vi "send Ack.vi"(8 "error in":errorcluster, 10 "State Change?":bool, 11 "EF20 in":refnum<class "EF20.lvclass">) -> (0 "error out":errorcluster, 3 "EF20 out":refnum<class "EF20.lvclass">)   [LabVIEW 2018, in "EF20.lvlib" / "EF20.lvclass"]
uses:
  EF20.lvclass
  EF20.lvclass/EF20.ctl
  Custom Controls/EF20 Message Type.ctl
  EF20.lvlib
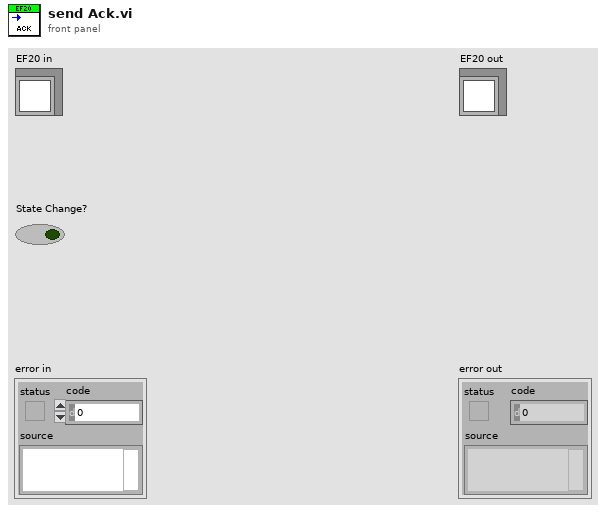
[diagram p1: front panel]
types:
  T1 = typedef "EF20.lvlib/EF20 Message Type.ctl" = u8
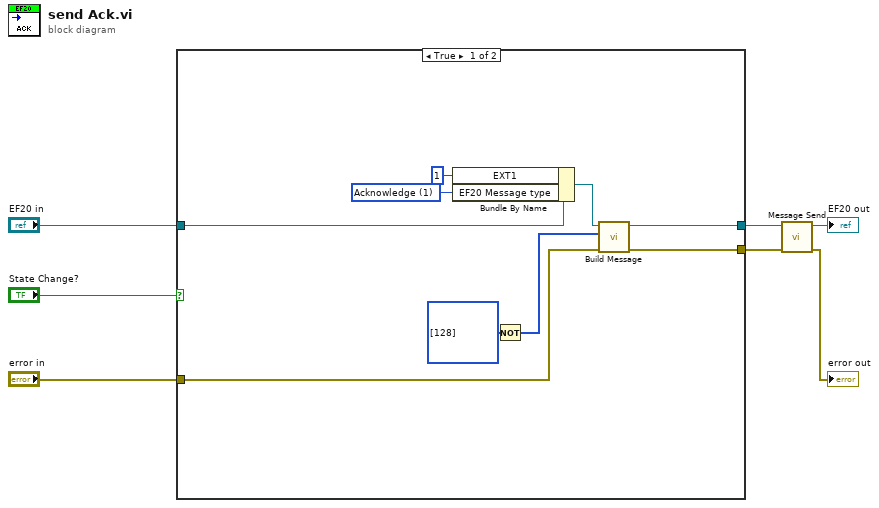
[diagram p0: block diagram]
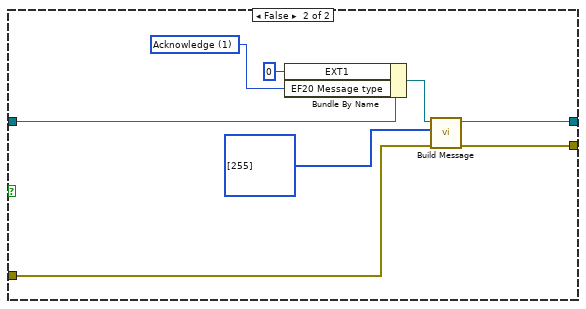
[diagram p2: hidden frame]
diagram:
  n1 = case shown="True" "State Change?" {
    tunnel: "EF20 in" -> [w16 w24]
    tunnel: [w15 w23] -> w5
    tunnel: [w14 w22] -> w2
    tunnel: "error in" -> [w13 w21]
    frame True {
      w12 = u8 1 items=["Update"=48, "Graph"=49, "Status"=50, "Parameter"=51, "Acknowledge"=1] ("EF20 Message type")
      n2 = Bundle By Name(cluster=w16, "EXT1"=u8 1, "EF20 Message type"=w12) -> (w11:refnum<class "EF20.lvclass">)
      n3 = Not(x=u8[] [128] ("Data to Send")) -> (.not. x?=w8:u8[])
      n4 = call "Build Message.vi"("error in (no error)"=w13, "Data to Send"=w8, "EF20 in"=w11) -> ("error out"=w14:errorcluster, "EF20 out"=w15:refnum<class "EF20.lvclass">)  [unwired: 7 in]
    }
    frame False {
      w17 = T1 1 items=["Update"=48, "Graph"=49, "Status"=50, "Parameter"=51, "Acknowledge"=1] ("EF20 Message type")
      n5 = Bundle By Name(cluster=w24, "EXT1"=u8 0, "EF20 Message type"=w17) -> (w20:refnum<class "EF20.lvclass">)
      n6 = call "Build Message.vi"("error in (no error)"=w21, "Data to Send"=u8[] [255], "EF20 in"=w20) -> ("error out"=w22:errorcluster, "EF20 out"=w23:refnum<class "EF20.lvclass">)  [unwired: 7 in]
    }
  }
  n7 = call "Message Send.vi"("error in"=w2, "EF20 in"=w5) -> ("error out"=→"error out":errorcluster, "EF20 out"=→"EF20 out":refnum<class "EF20.lvclass">)  [unwired: 8 in]
